vi "Gunsim Vision Adapter.vi"(1 "Other Constants":T1={"Ball Diameter(in)"=10.0, "Air Density(g/in^3)"=0.02, "Drag coefficient"=0.5, "Ball Mass(g)"=300.0, "gravity(in/s^2)"=-386.09, "Minimum Goal Height(in)"=90.0, "Maximum Goal Height(in)"=104.0}, 2 "cluster in":T3) -> (0 "cluster out":T2)   [LabVIEW 2015]
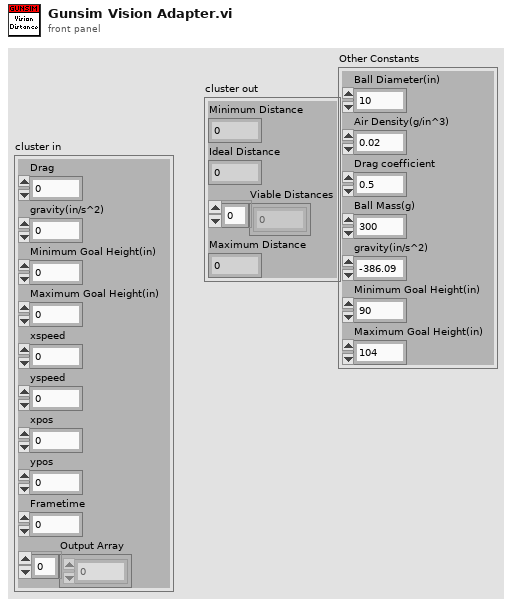
[diagram p1: front panel]
types:
  T1 = cluster{"Ball Diameter(in)":dbl, "Air Density(g/in^3)":dbl, "Drag coefficient":dbl, "Ball Mass(g)":dbl, "gravity(in/s^2)":dbl, "Minimum Goal Height(in)":dbl, "Maximum Goal Height(in)":dbl}
  T2 = cluster{"Minimum Distance":dbl, "Ideal Distance":dbl, "Viable Distances":dbl[], "Maximum Distance":dbl}
  T3 = cluster{"Drag":dbl, "gravity(in/s^2)":dbl, "Minimum Goal Height(in)":dbl, "Maximum Goal Height(in)":dbl, "xspeed":dbl, "yspeed":dbl, "xpos":dbl, "ypos":dbl, "Frametime":dbl, "Output Array":dbl[]}
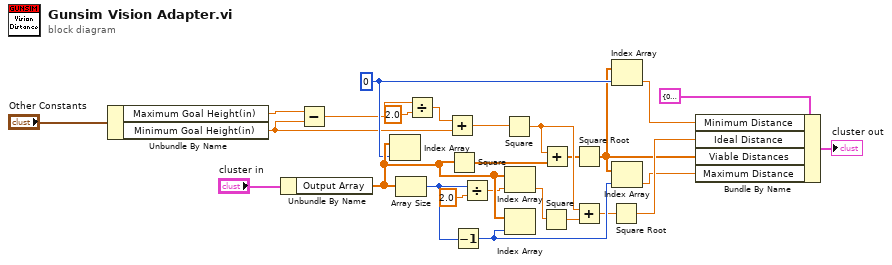
[diagram p0: block diagram]
diagram:
  w18 = 0 ("index")
  n1 = Unbundle By Name("Other Constants") -> ("Maximum Goal Height(in)"=w6:dbl, "Minimum Goal Height(in)"=w2:dbl)
  n2 = Unbundle By Name("cluster in") -> ("Output Array"=w26:dbl[])
  n3 = Subtract(x=w6, y=w2) -> (x-y=w4:dbl)
  n4 = Index Array(array=w26, index=w18) -> ()  [unwired: 1 out]
  n5 = Array Size(array=w26) -> (size(s)=w22:i32)
  n6 = Divide(x=w4, y=2.0) -> (x/y=w3:dbl)
  n7 = Add(x=w3, y=w2) -> (x+y=w1:dbl)
  n8 = Square(x=w26) -> (x^2=w14:dbl[])
  n9 = Decrement(x=w22) -> (x-1=w19:i32)
  n10 = Divide(x=w22, y=2.0) -> (x/y=w21:dbl)
  n11 = Square(x=w1) -> (x^2=w15:dbl)
  n12 = Index Array(array=w26, index=w21) -> (element=w23:dbl)
  n13 = Index Array(array=w26, index=w19) -> ()  [unwired: 1 out]
  n14 = Square(x=w23) -> (x^2=w12:dbl)
  n15 = Add(x=w15, y=w14) -> (x+y=w13:dbl[])
  n16 = Square Root(x=w13) -> (sqrt(x)=w16:dbl[])
  n17 = Add(x=w15, y=w12) -> (x+y=w11:dbl)
  n18 = Square Root(x=w11) -> (sqrt(x)=w24:dbl)
  n19 = Index Array(array=w16, index=w18) -> (element=w9:dbl)
  n20 = Index Array(array=w16, index=w19) -> (element=w10:dbl)
  n21 = Bundle By Name(cluster=T2 {"Minimum Distance"=0.0, "Ideal Distance"=0.0, "Viable Distances"=[], "Maximum Distance"=0.0} ("input cluster"), "Minimum Distance"=w9, "Ideal Distance"=w24, "Viable Distances"=w16, "Maximum Distance"=w10) -> (→"cluster out":T2)
